vi "DataInit.vi"(8 "error in (no error)":errorcluster, 11 "ClusterIN":T1) -> (0 "error out":errorcluster, 3 "ClusterOUT":T1)   [LabVIEW 2021]
uses:
  TypeDef/InitCluster.ctl
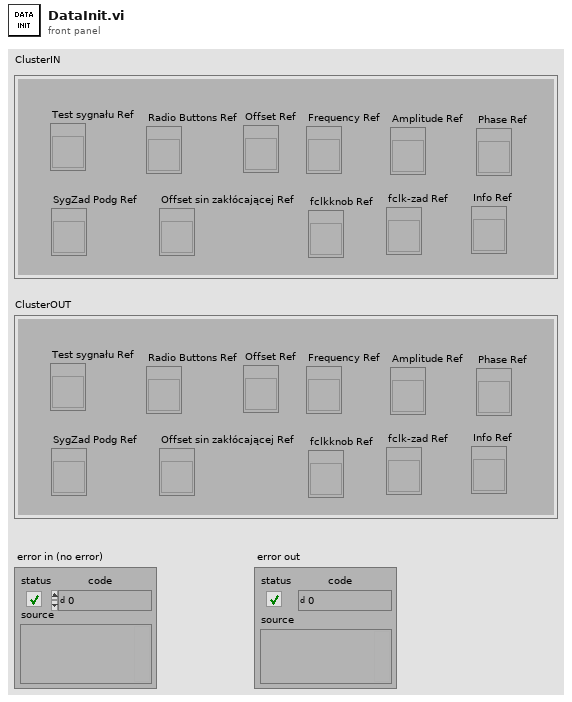
[diagram p1: front panel]
types:
  T1 = typedef "InitCluster.ctl" = cluster{"Offset Ref":refnum<vi>, "Frequency Ref":refnum<vi>, "Amplitude Ref":refnum<vi>, "Phase Ref":refnum<vi>, "SygZad Podg Ref":refnum<vi>, "Test sygnału Ref":refnum<vi>, "Radio Buttons Ref":refnum<vi>, "Offset sin zakłócającej Ref":refnum<vi>, "fclkknob Ref":refnum<vi>, "fclk-zad Ref":refnum<vi>, "Info Ref":refnum<vi>}
  T2 = enum8{"Enabled", "Disabled", "Disabled and Grayed Out"}
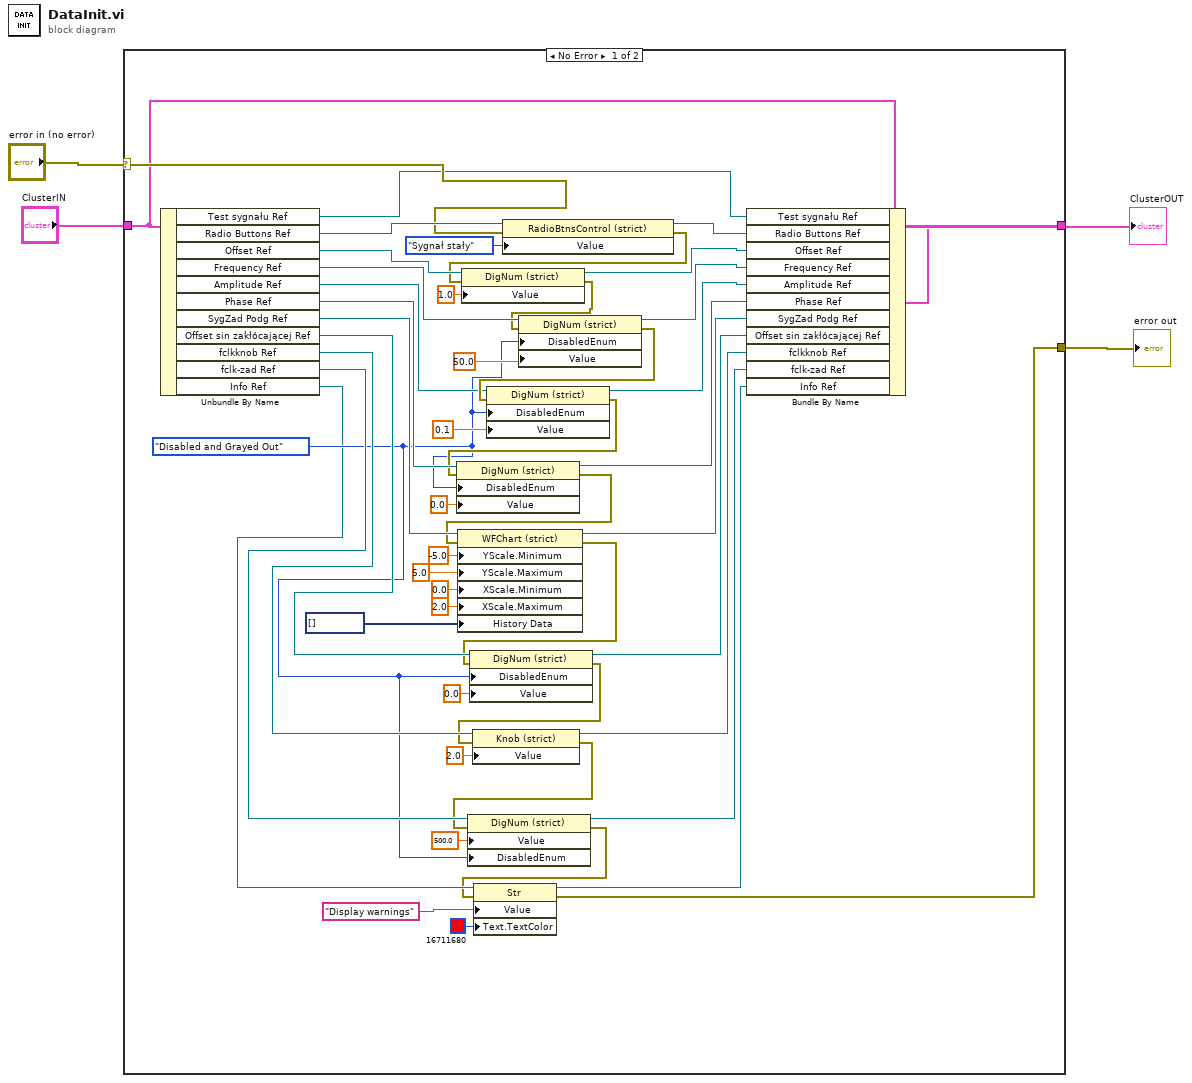
[diagram p0: block diagram]
diagram:
  n1 = case shown="No Error" "error in (no error)" {
    selector: "error in (no error)" -> [w27 w55]
    tunnel: "ClusterIN" -> [w11 w56]
    tunnel: [w12 w55] -> w2
    tunnel: [w38 w56] -> w1
    frame No Error {
      w16 = T2."Disabled and Grayed Out" ("Disabled")
      n2 = Unbundle By Name(w11) -> ("Test sygnału Ref"=w26:refnum<vi>, "Radio Buttons Ref"=w54:refnum<vi>, "Offset Ref"=w52:refnum<vi>, "Frequency Ref"=w49:refnum<vi>, "Amplitude Ref"=w46:refnum<vi>, "Phase Ref"=w45:refnum<vi>, "SygZad Podg Ref"=w37:refnum<vi>, "Offset sin zakłócającej Ref"=w25:refnum<vi>, "fclkknob Ref"=w22:refnum<vi>, "fclk-zad Ref"=w21:refnum<vi>, "Info Ref"=w15:refnum<vi>)
      n3 = property class="RadioBtnsControl (strict)"(reference=w54, error in=w27, "Value"=enum32{"Sygnał przemienny", "Sygnał stały"}."Sygnał stały") -> (reference out=w43:refnum<vi>, error out=w50:errorcluster)
      n4 = property class="DigNum (strict)"(reference=w52, error in=w50, "Value"=1.0) -> (reference out=w42:refnum<vi>, error out=w48:errorcluster)
      n5 = property class="DigNum (strict)"(reference=w49, error in=w48, "DisabledEnum"=w16, "Value"=50.0) -> (reference out=w41:refnum<vi>, error out=w47:errorcluster)
      n6 = property class="DigNum (strict)"(reference=w46, error in=w47, "DisabledEnum"=w16, "Value"=0.1) -> (reference out=w40:refnum<vi>, error out=w44:errorcluster)
      n7 = property class="DigNum (strict)"(reference=w45, error in=w44, "DisabledEnum"=w16, "Value"=0.0) -> (reference out=w39:refnum<vi>, error out=w36:errorcluster)
      n8 = property class="WFChart (strict)"(reference=w37, error in=w36, "YScale.Minimum"=-5.0 ("Y Scale.Range:Minimum"), "YScale.Maximum"=5.0 ("Y Scale.Range:Maximum"), "XScale.Minimum"=0.0 ("X Scale.Range:Minimum"), "XScale.Maximum"=2.0 ("X Scale.Range:Maximum"), "History Data"=dynamicdata[] []) -> (reference out=w10:refnum<vi>, error out=w24:errorcluster)
      n9 = property class="DigNum (strict)"(reference=w25, error in=w24, "DisabledEnum"=w16, "Value"=0.0) -> (reference out=w9:refnum<vi>, error out=w20:errorcluster)
      n10 = property class="Knob (strict)"(reference=w22, error in=w20, "Value"=2.0) -> (reference out=w8:refnum<vi>, error out=w19:errorcluster)
      n11 = property class="DigNum (strict)"(reference=w21, error in=w19, "Value"=500.0, "DisabledEnum"=w16) -> (reference out=w7:refnum<vi>, error out=w14:errorcluster)
      n12 = property class="Str"(reference=w15, error in=w14, "Value"="Display warnings", "Text.TextColor"=u32 16711680 ("Text.Text Colors:Text Color")) -> (reference out=w6:refnum<vi>, error out=w12:errorcluster)
      n13 = Bundle By Name(cluster=w11, "Test sygnału Ref"=w26, "Radio Buttons Ref"=w43, "Offset Ref"=w42, "Frequency Ref"=w41, "Amplitude Ref"=w40, "Phase Ref"=w39, "SygZad Podg Ref"=w10, "Offset sin zakłócającej Ref"=w9, "fclkknob Ref"=w8, "fclk-zad Ref"=w7, "Info Ref"=w6) -> (w38:T1)
    }
    frame Error {
    }
  }
  "ClusterOUT" <- w1
  "error out" <- w2
